vi "display.vi"(8 "error in (no error)":errorcluster, 11 "ModelDuck in":refnum<class "ModelDuck.lvclass">) -> (0 "error out":errorcluster, 2 "State":string, 3 "ModelDuck out":refnum<class "ModelDuck.lvclass">)   [LabVIEW 2013, in "ModelDuck.lvclass"]
uses:
  ModelDuck.lvclass
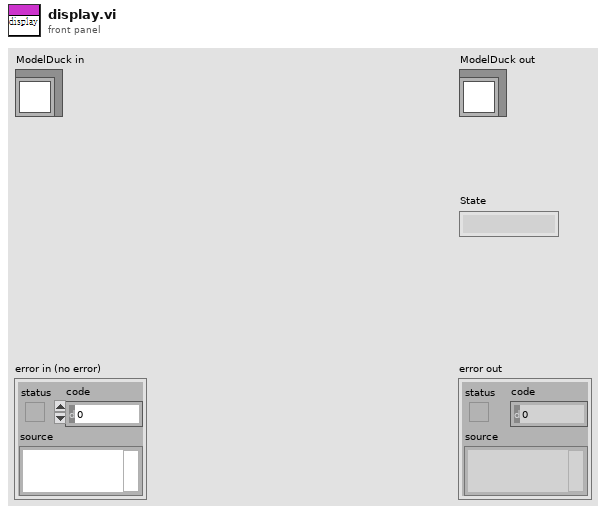
[diagram p1: front panel]
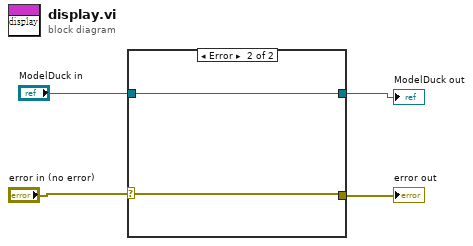
[diagram p0: block diagram]
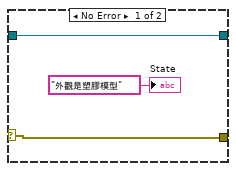
[diagram p2: hidden frame]
diagram:
  n1 = case shown="Error" "error in (no error)" {
    selector: "error in (no error)" -> [w6 w8]
    tunnel: [w6 w8] -> w3
    tunnel: [w5 w9] -> w2
    tunnel: "ModelDuck in" -> [w5 w9]
    frame No Error {
      "State" <- "外觀是塑膠模型" ("State")
    }
    frame Error {
    }
  }
  "error out" <- w3
  "ModelDuck out" <- w2
